vi "Display Value.vi"() -> ()   [LabVIEW 2023]
doc: "This vi reads the stored DVR reference and displays the data."
uses:
  Controls/StoreRef.ctl
panel:
  out "data value":dbl
  out "error out":errorcluster
  in  "error in (no error)":errorcluster
  in  "Display":bool
  in  "Stop":bool
  # "Instructions:\n\n-> Run the Vi\n-> Make sure DVR Creater.vi was running\n-> Press Get Value button to display data in indicator.\n-> Press STOP button to stop the running vi."
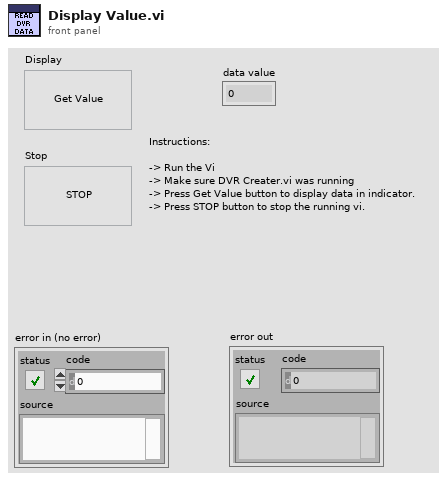
[diagram p1: front panel]
types:
  T1 = typedef "StoreRef.ctl" = enum16{"Store Ref", "Get Ref"}
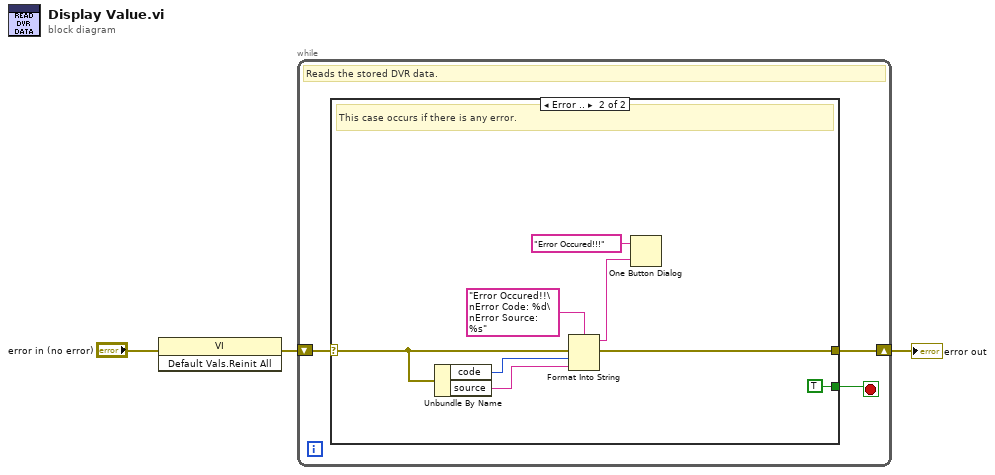
[diagram p0: block diagram]
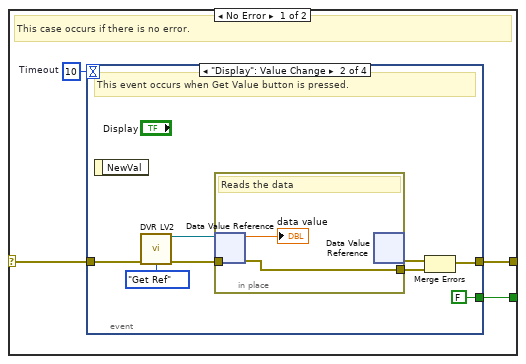
[diagram p2: hidden frame]
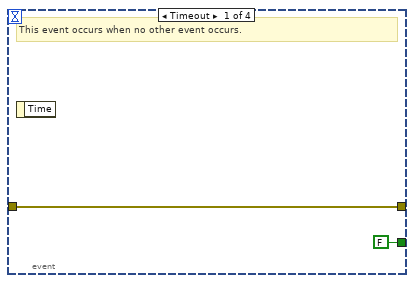
[diagram p3: hidden frame]
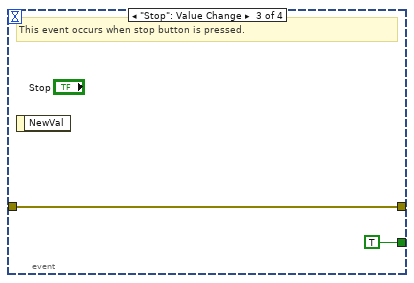
[diagram p4: hidden frame]
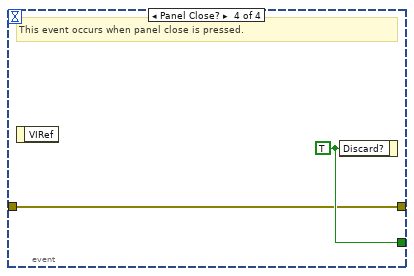
[diagram p5: hidden frame]
diagram:
  n1 = invoke class="VI" method="Default Vals.Reinit All"(error in="error in (no error)") -> (error out=w1:errorcluster)  [unwired: 2 in, 2 out]
  n2 = while {
    shift-right: [w5] -> w2
    shift-left: w1 -> [w6]
    stop <- w4 stop-if-true
    # "Reads the stored DVR data."
    n3 = case shown="Error .." w6 {
      selector: w6 -> [w9 w30]
      tunnel: [w8 w32] -> w5
      tunnel: [w7 TRUE ("Discard?")] -> w4
      frame No Error {
        w10 = 10  # Timeout
        # "This case occurs if there is no error."
        n4 = event shown="[1] \"Display\": Value Change" {
          selector: _ -> [_ _ _ _]
          dyn-events: _ -> [_ _ _ _]
          timeout: w10 -> [_ _ _ _]
          tunnel: w9 -> [w12 w20 w24 w25]
          tunnel: [w12 w13 w24 w25] -> w8
          tunnel: [FALSE ("Discard?") FALSE ("Discard?") TRUE w26] -> w7
          event Timeout {
            # "This event occurs when no other event occurs."
            n5 = event-data() -> ()  [unwired: 1 in, 1 out]
          }
          event "Display": Value Change {
            # "This event occurs when Get Value button is pressed."
            n6 = event-data() -> ()  [unwired: 1 in, 1 out]
            n7 = call "DVR LV2.vi"("error in (no error)"=w20, "Operation"=StoreRef."Get Ref") -> ("Data Value Reference Out"=w18:refnum<data-value>, "error out"=w19:errorcluster)  [unwired: 12 in]
            n8 = in-place {
              in-place-border: w19 -> [_]
              in-place-border: [w21] -> w14
              # "Reads the data"
              n9 = in-place-dvr #1(w18) -> (→"data value":dbl, w21:errorcluster)
              n10 = in-place-dvr #1() -> (w15:errorcluster)  [unwired: 1 in, 1 out]
            }
            n11 = Merge Errors(w15, w14) -> (w13:errorcluster)
          }
          event "Stop": Value Change {
            # "This event occurs when stop button is pressed."
            n12 = event-data() -> ()  [unwired: 1 in, 1 out]
          }
          event Panel Close? {
            w26 = TRUE ("Discard?")
            # "This event occurs when panel close is pressed."
            n13 = event-data() -> ()  [unwired: 1 in, 1 out]
            n14 = event-data("Discard?"=w26) -> ()  [unwired: 1 in, 1 out]
          }
        }
      }
      frame Error {
        # "This case occurs if there is any error."
        n15 = Unbundle By Name(w30) -> ("code"=w29:i32, "source"=w28:string)
        n16 = Format Into String(format string="Error Occured!!\nError Code: %d\nError Source: %s", error in=w30, w29, w28) -> (resulting string=w27:string, error out=w32:errorcluster)  [unwired: 1 in]
        n17 = One Button Dialog(message="Error Occured!!!", button name ("OK")=w27) -> ()  [unwired: 1 out]
      }
    }
  }
  "error out" <- w2
